vi "Write Distributional Statistics.vi"(8 "error in (no error)":errorcluster, 10 "Distributional Statistics":T1, 11 "DROPBEAR_Model_Updating in":refnum<class "DROPBEAR_Model_Updating.lvclass">) -> (0 "error out":errorcluster, 3 "DROPBEAR_Model_Updating out":refnum<class "DROPBEAR_Model_Updating.lvclass">)   [LabVIEW 2021, in "DROPBEAR_Model_Updating.lvclass"]
uses:
  DROPBEAR_Model_Updating.lvclass
  Online_Statistic/Online_Statistic.lvclass
  DROPBEAR_Model_Updating.lvclass/DROPBEAR_Model_Updating.ctl
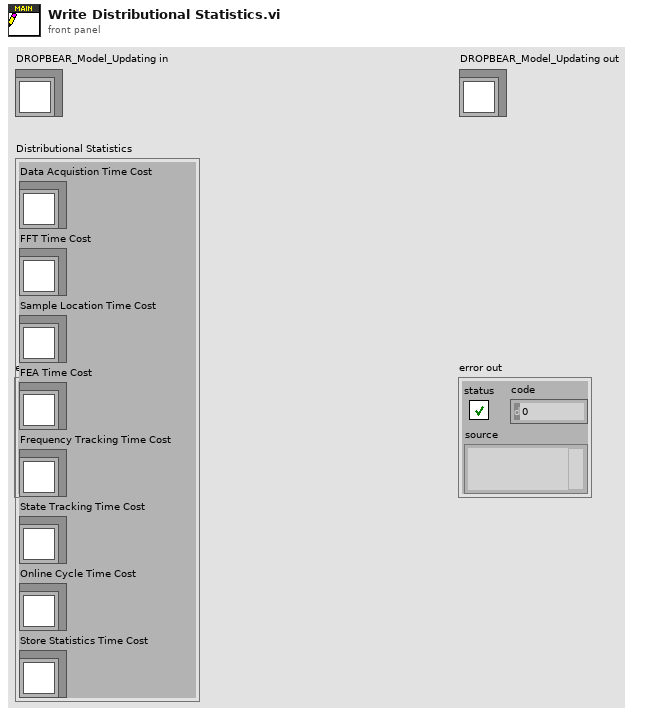
[diagram p1: front panel]
types:
  T1 = cluster{"Data Acquistion Time Cost":refnum<class "Online_Statistic.lvclass">, "FFT Time Cost":refnum<class "Online_Statistic.lvclass">, "Frequency Tracking Time Cost":refnum<class "Online_Statistic.lvclass">, "Sample Location Time Cost":refnum<class "Online_Statistic.lvclass">, "FEA Time Cost":refnum<class "Online_Statistic.lvclass">, "State Tracking Time Cost":refnum<class "Online_Statistic.lvclass">, "Online Cycle Time Cost":refnum<class "Online_Statistic.lvclass">, "Store Statistics Time Cost":refnum<class "Online_Statistic.lvclass">}
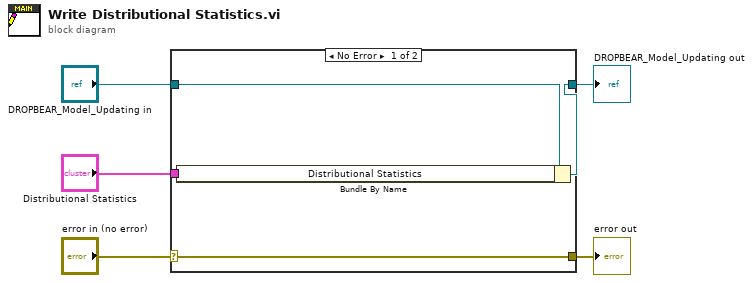
[diagram p0: block diagram]
diagram:
  n1 = case shown="No Error" "error in (no error)" {
    selector: "error in (no error)" -> [w9 w10]
    tunnel: [w9 w10] -> w4
    tunnel: [w7 w11] -> w2
    tunnel: "DROPBEAR_Model_Updating in" -> [w8 w11]
    tunnel: "Distributional Statistics" -> [w6 _]
    frame No Error {
      n2 = Bundle By Name(cluster=w8, "Distributional Statistics"=w6) -> (w7:refnum<class "DROPBEAR_Model_Updating.lvclass">)
    }
    frame Error {
    }
  }
  "error out" <- w4
  "DROPBEAR_Model_Updating out" <- w2
